vi "ep_Flicker Block3b.vi"(0 "filtered voltage":dbl[](array[numeric]), 1 "init":bool, 5 "voltage system":enum16{"120 V", "230 V"}(ring), 9 "input sampling rate":dbl=400.0) -> (4 "weighted voltage fluctuation":dbl[](array[numeric]))   [LabVIEW 2011, in "NI_EP_Power Quality.lvlib"]
doc: "This VI represents the second filter (of block 3 according IEC 61000-4-15), which is a weighting filter block that simulates the frequency response to sinusoidal voltage fluctuations of a coiled filament gas-filled lamp (60 W – 230 V) combined with the human visual system. The response function is based on the perceptibility threshold found at each frequency by 50 % of the persons tested."
uses:
  <vilib>/addons/Electrical Power/PQ/NI_EP_Power Quality.lvlib
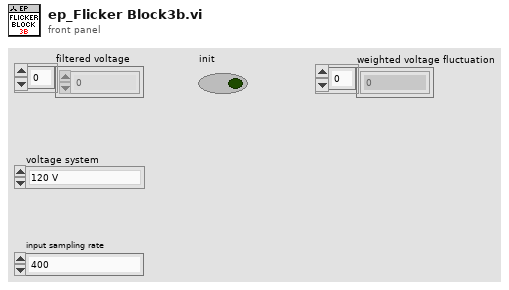
[diagram p1: front panel]
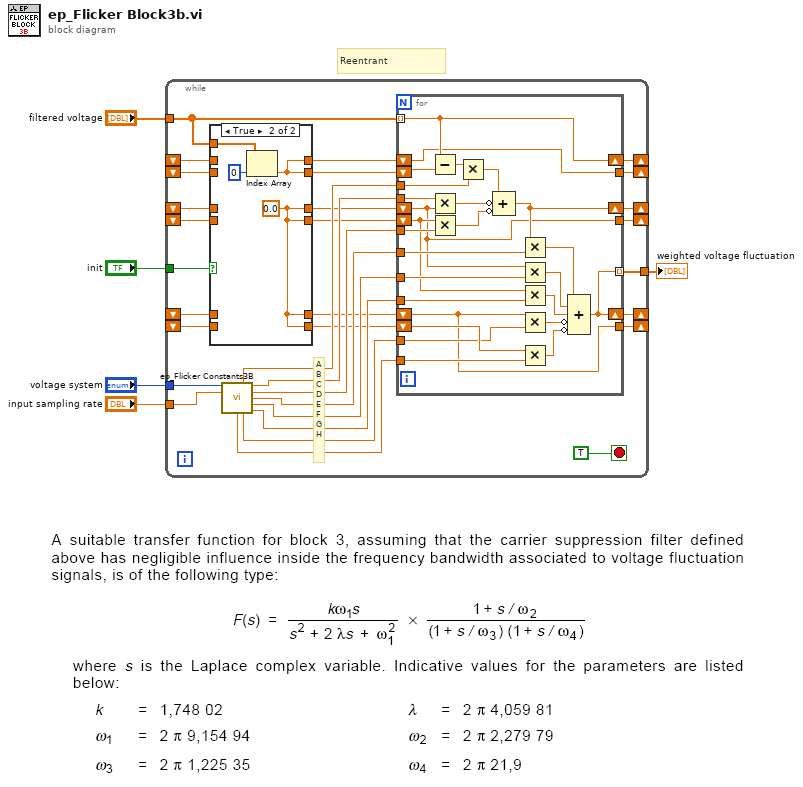
[diagram p0: block diagram]
diagram:
  # "Reentrant"
  n1 = while {
    tunnel: "init" -> [w7]
    shift-left: _ -> [w12]
    shift-right: [w22] -> _
    shift-left: _ -> [w16]
    shift-right: [w35] -> _
    shift-left: _ -> [w8]
    shift-right: [w36] -> _
    tunnel: "filtered voltage" -> [w6]
    tunnel: [w23] -> w5
    tunnel: "voltage system" -> [w33]
    tunnel: "input sampling rate" -> [w32]
    shift-right: [w20] -> _
    shift-left: _ -> [w9]
    shift-right: [w19] -> _
    shift-left: _ -> [w13]
    shift-right: [w18] -> _
    shift-left: _ -> [w10]
    stop <- TRUE stop-if-true
    # "A\nB\nC\nD\nE\nF\nG\nH"
    n2 = case shown="True" w7 {
      tunnel: [w38 w46] -> w37
      tunnel: [w41 w45] -> w21
      tunnel: w6 -> [_ w44]
      tunnel: [w39 w46] -> w17
      tunnel: w16 -> [w43 _]
      tunnel: [w43 w45] -> w15
      tunnel: [w42 w45] -> w14
      tunnel: w13 -> [w42 _]
      tunnel: w12 -> [w41 _]
      tunnel: [w40 w45] -> w11
      tunnel: w10 -> [w40 _]
      tunnel: w9 -> [w39 _]
      tunnel: w8 -> [w38 _]
      frame False {
      }
      frame True {
        w45 = 0.0
        n3 = Index Array(array=w44, index=0) -> (element=w46:dbl)
      }
    }
    n4 = call <vilib>:"ep_Flicker Constants3B.vi"("voltage system"=w33, "input sampling rate"=w32) -> ("A"=w31:dbl, "B"=w30:dbl, "C"=w29:dbl, "D"=w28:dbl, "E"=w27:dbl, "H"=w24:dbl, "G"=w25:dbl, "F"=w26:dbl)  [unwired: 6 in]
    n5 = for {
      shift-right: [w70] -> w36
      shift-left: w37 -> [w50]
      shift-left: w17 -> [w73]
      shift-right: [w57] -> w35
      shift-left: w15 -> [w49]
      shift-left: w14 -> [w62]
      tunnel: w6 -> [w70] mode=indexing
      tunnel: w30 -> [w71]
      tunnel: w31 -> [w61]
      tunnel: w29 -> [w69]
      tunnel: w28 -> [w68]
      shift-right: [w54] -> w22
      shift-left: w21 -> [w48]
      shift-left: w11 -> [w67]
      tunnel: [w54] -> w23 mode=indexing
      tunnel: w27 -> [w66]
      tunnel: w26 -> [w65]
      tunnel: w25 -> [w64]
      tunnel: w24 -> [w63]
      tunnel: [w50] -> w20
      tunnel: [w49] -> w19
      tunnel: [w48] -> w18
      n6 = Subtract(x=w70, y=w73) -> (x-y=w72:dbl)
      n7 = Multiply(x=w71, y=w49) -> (x*y=w59:dbl)
      n8 = Multiply(x=w62, y=w69) -> (x*y=w58:dbl)
      n9 = Multiply(x=w72, y=w61) -> (x*y=w60:dbl)
      n10 = Compound Arithmetic op=ADD(w60, invert w59, invert w58) -> (w57:dbl)
      n11 = Multiply(x=w57, y=w68) -> (x*y=w53:dbl)
      n12 = Multiply(x=w49, y=w66) -> (x*y=w52:dbl)
      n13 = Multiply(x=w62, y=w65) -> (x*y=w51:dbl)
      n14 = Multiply(x=w48, y=w64) -> (x*y=w56:dbl)
      n15 = Multiply(x=w67, y=w63) -> (x*y=w55:dbl)
      n16 = Compound Arithmetic op=ADD(w53, w52, w51, invert w56, invert w55) -> (w54:dbl)
    }
  }
  "weighted voltage fluctuation" <- w5
